vi "Vision Enables.vi"(1 "enable/disable":bool) -> ()   [LabVIEW 2013]
uses:
  typedefs/fg_typedef.ctl
  typedefs/Vision/vision enable.ctl
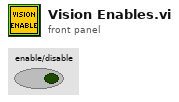
[diagram p1: front panel]
types:
  T1 = typedef "vision enable.ctl" = enum16{"Enable", "Disable", "Stop"}
  T2 = typedef "fg_typedef.ctl" = enum16{"Get", "Set"}
  T3 = cluster{"Left":dbl, "Top":dbl, "Right":dbl, "Bottom":dbl, "Target CoM X":dbl, "Target CoM Y":dbl}
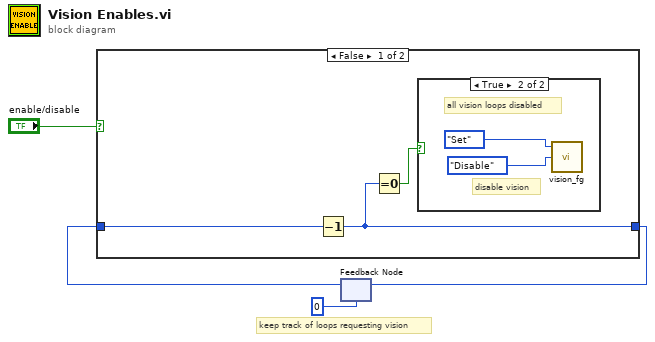
[diagram p0: block diagram]
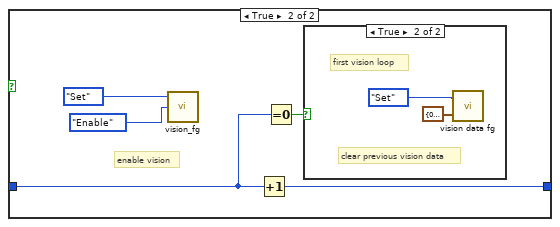
[diagram p3: hidden frame]
diagram:
  # "keep track of loops requesting vision"
  n1 = feedback #1(0) -> (w2:i32)
  n2 = case shown="False" "enable/disable" {
    tunnel: w2 -> [w7 w12]
    tunnel: [w6 w14] -> w1
    frame False {
      n3 = Decrement(x=w7) -> (x-1=w6:i32)
      n4 = Equal To 0?(x=w6) -> (x = 0?=w5:bool)
      n5 = case shown="True" w5 {
        frame False {
        }
        frame True {
          # "all vision loops disabled"
          # "disable vision"
          n6 = call "vision_fg.vi"("Action"=vision_enable."Disable", "Menu"=fg_typedef."Set" ("Enum")) -> ()  [unwired: 1 in, 2 out]
        }
      }
    }
    frame True {
      # "enable vision"
      n7 = call "vision_fg.vi"("Action"=vision_enable."Enable", "Menu"=fg_typedef."Set" ("Enum")) -> ()  [unwired: 1 in, 2 out]
      n8 = Increment(x=w12) -> (x+1=w14:i32)
      n9 = Equal To 0?(x=w12) -> (x = 0?=w13:bool)
      n10 = case shown="True" w13 {
        frame False {
          # "already enabled"
        }
        frame True {
          # "first vision loop"
          # "clear previous vision data"
          n11 = call "vision data fg.vi"("Input"=T3 {"Left"=0.0, "Top"=0.0, "Right"=0.0, "Bottom"=0.0, "Target CoM X"=0.0, "Target CoM Y"=0.0}, "Menu"=fg_typedef."Set" ("Enum")) -> ()  [unwired: 1 out]
        }
      }
    }
  }
  n12 = feedback-in #1(w1) -> ()
